vi "Elapsed Time.vi"() -> ()   [LabVIEW 2010]
doc: "This VI demonstrates the differences between the timing functions."
panel:
  in  "stop":bool
  out "Total Elapsed Time":u32
  out "Time Between Iterations":u32
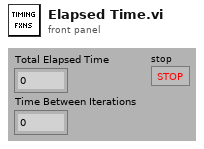
[diagram p1: front panel]
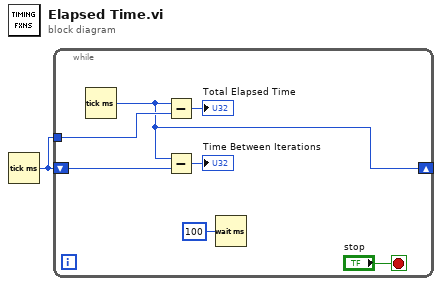
[diagram p0: block diagram]
diagram:
  n1 = Tick Count (ms)() -> (millisecond timer value=w1:u32)
  n2 = while {
    shift-right: [w5] -> _
    shift-left: w1 -> [w8]
    tunnel: w1 -> [w6]
    stop <- "stop" stop-if-true
    n3 = Tick Count (ms)() -> (millisecond timer value=w5:u32)
    n4 = Subtract(x=w5, y=w6) -> (x-y=→"Total Elapsed Time":u32)
    n5 = Subtract(x=w5, y=w8) -> (x-y=→"Time Between Iterations":u32)
    n6 = Wait (ms)(milliseconds to wait=u32 100) -> ()  [unwired: 1 out]
  }
